vi "2020-TestCodeOnWindows.vi"() -> ()   [LabVIEW 2020]
panel:
  in  "error in":errorcluster
  out "error out":errorcluster
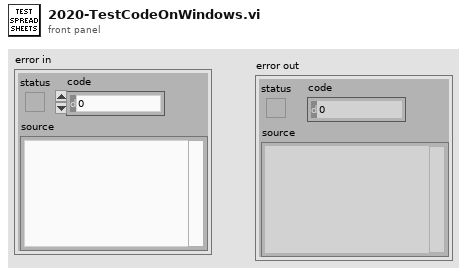
[diagram p1: front panel]
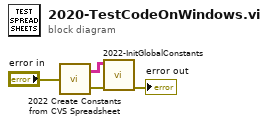
[diagram p0: block diagram]
diagram:
  n1 = call "2022 Create Constants from CVS Spreadsheet.vi"("error in"="error in") -> ("localConstantSpreadSheet"=w3:string[][], "error out"=w2:errorcluster)
  n2 = call "2022-InitGlobalConstants.vi"("error in (no error)"=w2, "localConstantSpreadSheet"=w3) -> ("error out"=→"error out":errorcluster)  [unwired: 9 in]
